vi "Init Events.vi"(8 "error in (no error)":errorcluster, 11 "VectoService in":refnum<class "VectoInfo.lvclass">) -> (0 "error out":errorcluster, 3 "VectoService out":refnum<class "VectoInfo.lvclass">)   [LabVIEW 2020, in "Vecto.lvlib" / "VectoInfo.lvclass"]
uses:
  VectoInfo.lvclass
  lv-promises/Promises/Promise/Promise.lvclass
  Incoming Events.ctl
  Connection Data.ctl
  Connection Info.ctl
  Connection Type.ctl
  Info Data.ctl
  Vecto Info.ctl
  Count Data.ctl
  VectoInfo.lvclass/VectoInfo.ctl
  Vecto.lvlib
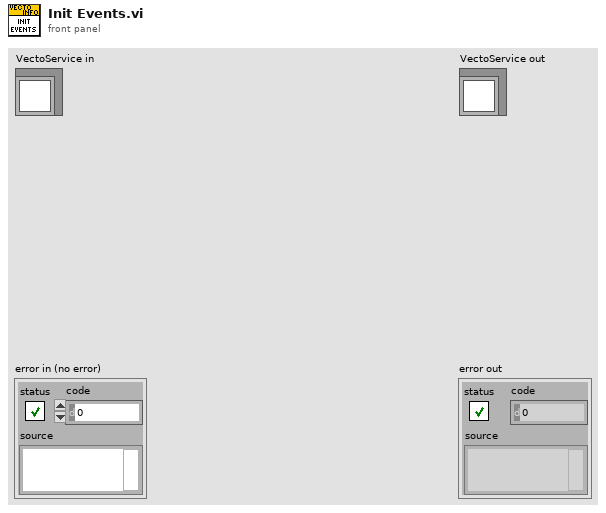
[diagram p1: front panel]
types:
  T1 = typedef "Vecto.lvlib/VectoInfo.lvclass/Count Data.ctl" = cluster{"Name":string, "Amount":i32}
  T2 = typedef "Vecto.lvlib/VectoInfo.lvclass/Info Data.ctl" = cluster{"Info":T3}
  T3 = typedef "Vecto.lvlib/Vecto Info.ctl" = cluster{"NodeID":i32, "IP":u32, "Connections":T4[]}
  T4 = typedef "Vecto.lvlib/Connection Info.ctl" = cluster{"Name":string, "Type":T5, "RXCount":i32, "TXCount":i32, "Connected":bool, "RemoteIP":u32, "RemotePort":u16, "LocalPort":u16, "Node ID":u32}
  T5 = typedef "Vecto.lvlib/Connection Type.ctl" = enum16{"TCP", "Telemetry", "Discovery", "HTTP"}
  T6 = typedef "Vecto.lvlib/VectoInfo.lvclass/Connection Data.ctl" = cluster{"Info":T4}
  T7 = typedef "Vecto.lvlib/VectoInfo.lvclass/Incoming Events.ctl" = cluster{"Request Info":refnum<user-event>, "Update Connection":refnum<user-event>, "Update Info":refnum<user-event>, "Close":refnum<user-event>, "Remove Connection":refnum<user-event>, "Add RX":refnum<user-event>, "Add TX":refnum<user-event>}
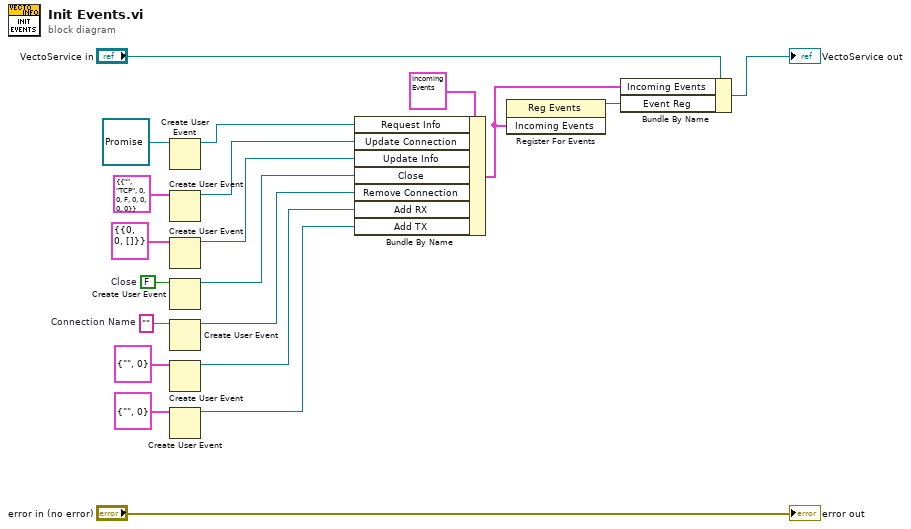
[diagram p0: block diagram]
diagram:
  w6 = ""  # Connection Name
  w8 = FALSE  # Close
  n1 = Create User Event(user event datatype=refnum<class "Promise.lvclass"> refnum ("Futures:Promise")) -> (user event=w18:refnum<user-event>)  [unwired: 1 in, 1 out]
  n2 = Create User Event(user event datatype=T6 {"Info"={"Name"="", "Type"=enum."TCP", "RXCount"=0, "TXCount"=0, "Connected"=FALSE, "RemoteIP"=0, "RemotePort"=0, "LocalPort"=0, "Node ID"=0}} ("Connection Data")) -> (user event=w12:refnum<user-event>)  [unwired: 1 in, 1 out]
  n3 = Create User Event(user event datatype=T2 {"Info"={"NodeID"=0, "IP"=0, "Connections"=[]}} ("Info Data")) -> (user event=w9:refnum<user-event>)  [unwired: 1 in, 1 out]
  n4 = Create User Event(user event datatype=w8) -> (user event=w7:refnum<user-event>)  [unwired: 1 in, 1 out]
  n5 = Create User Event(user event datatype=w6) -> (user event=w5:refnum<user-event>)  [unwired: 1 in, 1 out]
  n6 = Create User Event(user event datatype=T1 {"Name"="", "Amount"=0} ("Count Data")) -> (user event=w2:refnum<user-event>)  [unwired: 1 in, 1 out]
  n7 = Create User Event(user event datatype=T1 {"Name"="", "Amount"=0} ("Count Data")) -> (user event=w1:refnum<user-event>)  [unwired: 1 in, 1 out]
  n8 = Bundle By Name(cluster=T7 {"Request Info"=refnum, "Update Connection"=refnum, "Update Info"=refnum, "Close"=refnum, "Remove Connection"=refnum, "Add RX"=refnum, "Add TX"=refnum} ("Incoming Events"), "Request Info"=w18, "Update Connection"=w12, "Update Info"=w9, "Close"=w7, "Remove Connection"=w5, "Add RX"=w2, "Add TX"=w1) -> (w15:T7)
  n9 = register-events(w15) -> (reference out=w16:refnum<event-registration>)  [unwired: 2 in, 1 out]
  n10 = Bundle By Name(cluster="VectoService in", "Incoming Events"=w15, "Event Reg"=w16) -> (→"VectoService out":refnum<class "VectoInfo.lvclass">)
  "error out" <- "error in (no error)"
